vi "Get_Available_Flows.vi"(1 "Argument List":string[](array[string])) -> (0 "Available Flows":string[](array[string]))   [LabVIEW 2011]
doc: "This VI examines an argument list, determines the number of available flows (e.g., \"Flow1\", \"Flow2\", etc) and returns them in the form of a string array."
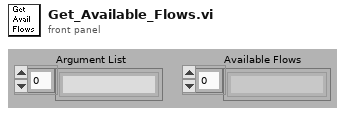
[diagram p1: front panel]
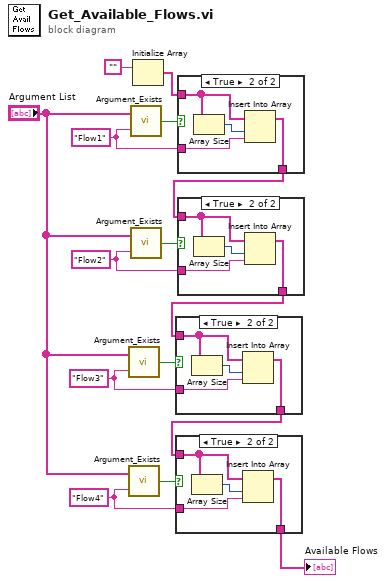
[diagram p0: block diagram]
diagram:
  w4 = "Flow4" ("Argument")
  w7 = "Flow3" ("Argument")
  w10 = "Flow2" ("Argument")
  w14 = "Flow1" ("Argument")
  n1 = call "Argument_Exists.vi"("Argument"=w7, "Argument List"="Argument List") -> ("Argument Exists"=w8:bool)
  n2 = call "Argument_Exists.vi"("Argument"=w4, "Argument List"="Argument List") -> ("Argument Exists"=w5:bool)
  n3 = call "Argument_Exists.vi"("Argument"=w14, "Argument List"="Argument List") -> ("Argument Exists"=w13:bool)
  n4 = call "Argument_Exists.vi"("Argument"=w10, "Argument List"="Argument List") -> ("Argument Exists"=w12:bool)
  n5 = Initialize Array("") -> (w11:string[])  [unwired: 1 out]
  n6 = case shown="True" w13 {
    tunnel: w14 -> [_ w20]
    tunnel: w11 -> [w16 w18]
    tunnel: [w16 w17] -> w9
    frame False {
    }
    frame True {
      n7 = Array Size(array=w18) -> (size(s)=w19:i32)
      n8 = Insert Into Array(array=w18, index=w19, new element=w20) -> (w17:string[])
    }
  }
  n9 = case shown="True" w12 {
    tunnel: w10 -> [_ w25]
    tunnel: w9 -> [w21 w23]
    tunnel: [w21 w22] -> w6
    frame False {
    }
    frame True {
      n10 = Array Size(array=w23) -> (size(s)=w24:i32)
      n11 = Insert Into Array(array=w23, index=w24, new element=w25) -> (w22:string[])
    }
  }
  n12 = case shown="True" w8 {
    tunnel: w7 -> [_ w30]
    tunnel: w6 -> [w26 w28]
    tunnel: [w26 w27] -> w3
    frame False {
    }
    frame True {
      n13 = Array Size(array=w28) -> (size(s)=w29:i32)
      n14 = Insert Into Array(array=w28, index=w29, new element=w30) -> (w27:string[])
    }
  }
  n15 = case shown="True" w5 {
    tunnel: w4 -> [_ w35]
    tunnel: w3 -> [w31 w33]
    tunnel: [w31 w32] -> w1
    frame False {
    }
    frame True {
      n16 = Array Size(array=w33) -> (size(s)=w34:i32)
      n17 = Insert Into Array(array=w33, index=w34, new element=w35) -> (w32:string[])
    }
  }
  "Available Flows" <- w1
